vi "command-status-ae.vi"(8 "Engine state":T2(ring), 10 "Add to complete":cluster{"Subsytem":T1, "Line #":i32}[](array[cluster]), 11 "Add to sent":cluster{"Subsytem":T1, "Line #":i32}[](array[cluster])) -> (2 "Complete":cluster{"Subsytem":T1, "Line #":i32}[](array[cluster]), 3 "Sent":cluster{"Subsytem":T1, "Line #":i32}[](array[cluster]))   [LabVIEW 2017, in "labview-standard-library.lvlib" / "automode-scripting.lvlib"]
uses:
  automode-scripting.lvlib
  type-defs/subsystems.ctl
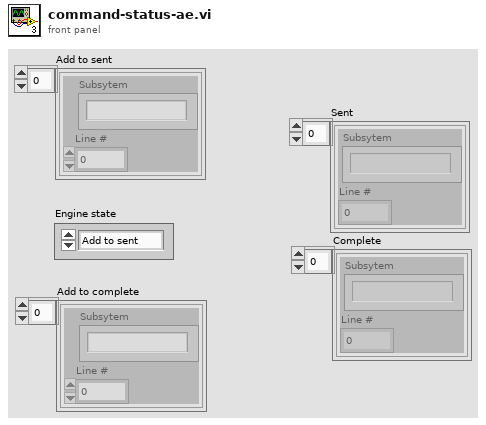
[diagram p1: front panel]
types:
  T1 = typedef "labview-standard-library.lvlib/automode-scripting.lvlib/subsystems.ctl" = string
  T2 = enum16{"Add to sent", "Add to complete", "Get arrays"}
  T3 = enum16{"Add to complete", "Add to sent", "Check"}
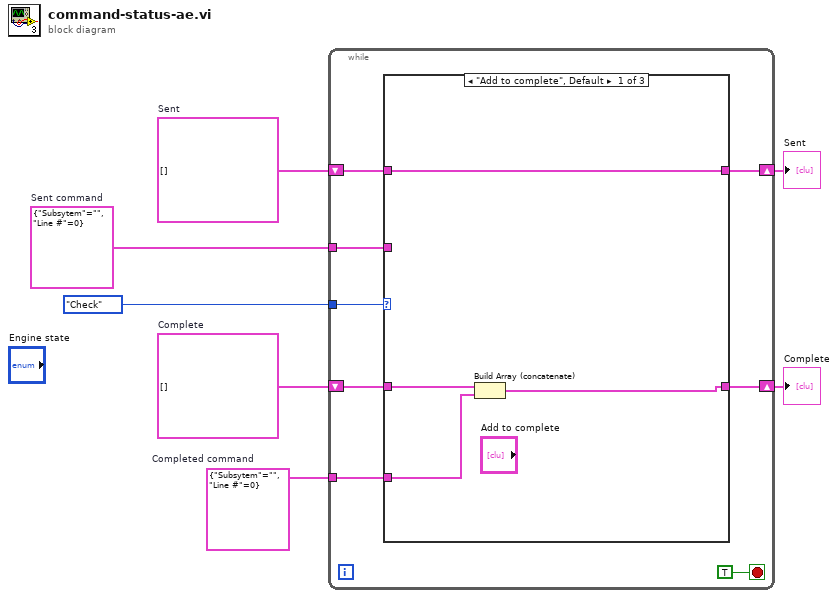
[diagram p0: block diagram]
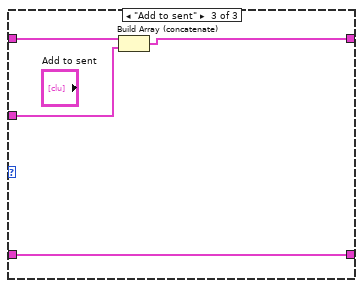
[diagram p3: hidden frame]
diagram:
  w4 = cluster{"Subsytem":T1, "Line #":i32} {"Subsytem"="", "Line #"=0}  # Completed command
  w3 = cluster{"Subsytem":T1, "Line #":i32} {"Subsytem"="", "Line #"=0}  # Sent command
  w6 = cluster{"Subsytem":T1, "Line #":i32}[] []  # Complete
  w7 = cluster{"Subsytem":T1, "Line #":i32}[] []  # Sent
  n1 = while {
    shift-right: [w10] -> w2
    shift-left: w7 -> [w13]
    shift-right: [w8] -> w1
    shift-left: w6 -> [w9]
    tunnel: T3."Check" -> [w14]
    tunnel: w4 -> [w12]
    tunnel: w3 -> [w11]
    stop <- TRUE stop-if-true
    n2 = case shown="\"Add to complete\", Default" w14 {
      tunnel: w13 -> [w19 w21 w25]
      tunnel: w12 -> [w17 _ _]
      tunnel: w11 -> [_ _ w24]
      tunnel: [w19 w21 w23] -> w10
      tunnel: w9 -> [w18 w20 w22]
      tunnel: [w16 w20 w22] -> w8
      frame "Add to complete", Default {
        n3 = Build Array (concatenate)(w18, w17) -> (w16:cluster{"Subsytem":T1, "Line #":i32}[])
      }
      frame "Check" {
      }
      frame "Add to sent" {
        n4 = Build Array (concatenate)(w25, w24) -> (w23:cluster{"Subsytem":T1, "Line #":i32}[])
      }
    }
  }
  "Sent" <- w2
  "Complete" <- w1
